vi "Read ADC UI.vi"(8 "error in (no error)":errorcluster, 11 "UI ACTOR in":refnum<class "UI ACTOR.lvclass">) -> (0 "error out":errorcluster, 3 "UI ACTOR out":refnum<class "UI ACTOR.lvclass">)   [LabVIEW 2020, in "UI ACTOR.lvlib" / "UI ACTOR.lvclass"]
uses:
  UI ACTOR.lvclass
  UI ACTOR.lvclass/UI ACTOR.ctl
  HAL/Proyecto-Final/Abstract/Serial Device/Serial Device.lvclass
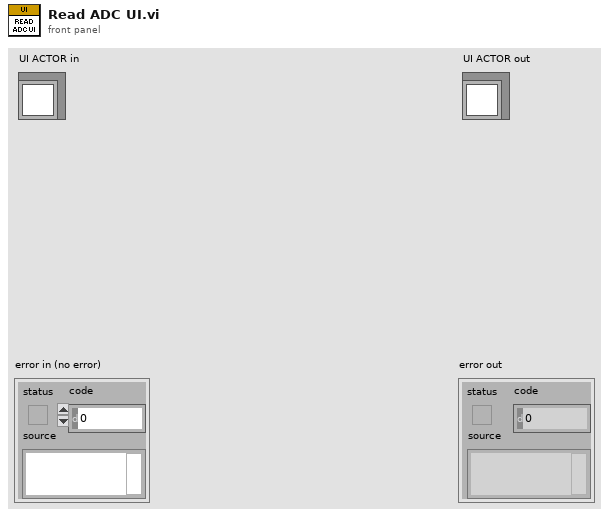
[diagram p1: front panel]
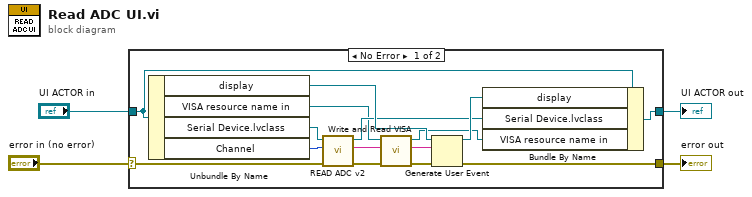
[diagram p0: block diagram]
diagram:
  n1 = case shown="No Error" "error in (no error)" {
    selector: "error in (no error)" -> [w17 w21]
    tunnel: [w14 w21] -> w3
    tunnel: [w12 w20] -> w1
    tunnel: "UI ACTOR in" -> [w13 w20]
    frame No Error {
      n2 = Unbundle By Name(w13) -> ("display"=w15:refnum<user-event>, "VISA resource name in"=w8:refnum<visa-resource-name>, "Serial Device.lvclass"=w19:refnum<class "Serial Device.lvclass">, "Channel"=w18:i32)
      n3 = call "READ ADC v2.vi"("error in (no error)"=w17, "Channel"=w18, "Serial Device in"=w19) -> ("error out"=w16:errorcluster, "Command  to send"=w7:string, "Serial Device out"=w10:refnum<class "Serial Device.lvclass">)  [unwired: 5 in, 1 out]
      n4 = call "Write and Read VISA.vi"("error in (no error)"=w16, "Command to Send"=w7, "VISA resource name in"=w8) -> ("error out"=w9:errorcluster, "Expected Response"=w5:string, "VISA resource name out"=w6:refnum<visa-resource-name>)  [unwired: 6 in]
      n5 = Generate User Event(user event=w15, event data cluster=w5, error in=w9) -> (user event out=w11:refnum<user-event>, error out=w14:errorcluster)  [unwired: 1 in]
      n6 = Bundle By Name(cluster=w13, "display"=w11, "Serial Device.lvclass"=w10, "VISA resource name in"=w6) -> (w12:refnum<class "UI ACTOR.lvclass">)
    }
    frame Error {
    }
  }
  "error out" <- w3
  "UI ACTOR out" <- w1
